vi "DSF.Engine.Timing.Increment.vi"(11 "Timing in":refnum<class "DSF.Engine.Timing.lvclass">) -> (3 "Timing out":refnum<class "DSF.Engine.Timing.lvclass">)   [LabVIEW 2017, in "DSF.Engine.lvlib" / "DSF.Engine.Timing.lvclass"]
uses:
  DSF.Engine.Timing.lvclass
  DSF.Engine.Timing.lvclass/DSF.Engine.Timing.ctl
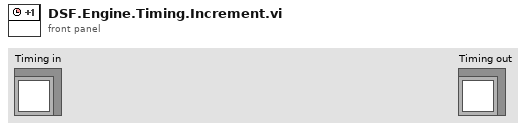
[diagram p1: front panel]
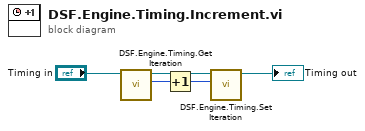
[diagram p0: block diagram]
diagram:
  n1 = call "DSF.Engine.Timing.Get Iteration.vi"("Timing in"="Timing in") -> ("Iteration"=w2:u64, "Timing out"=w4:refnum<class "DSF.Engine.Timing.lvclass">)  [unwired: 9 in]
  n2 = Increment(x=w2) -> (x+1=w1:u64)
  n3 = call "DSF.Engine.Timing.Set Iteration.vi"("Iteration"=w1, "Timing in"=w4) -> ("Timing out"=→"Timing out":refnum<class "DSF.Engine.Timing.lvclass">)  [unwired: 9 in]
